vi "superimpose_test.vi"() -> ()   [LabVIEW 2017]
uses:
  Vision.lvlib
panel:
  out "Image 2":T1(plugin-control)
  in  "Top Image":path=path "C:/Users/Caleb/Desktop/obama.jpg"
  in  "Y":i32=40
  in  "X":i32=20
  in  "Bottom Image":path=path "C:/Users/Caleb/Desktop/Screenshot 2021-05-22 162436.png"
  out "error out":errorcluster
  out "Image":T1(plugin-control)
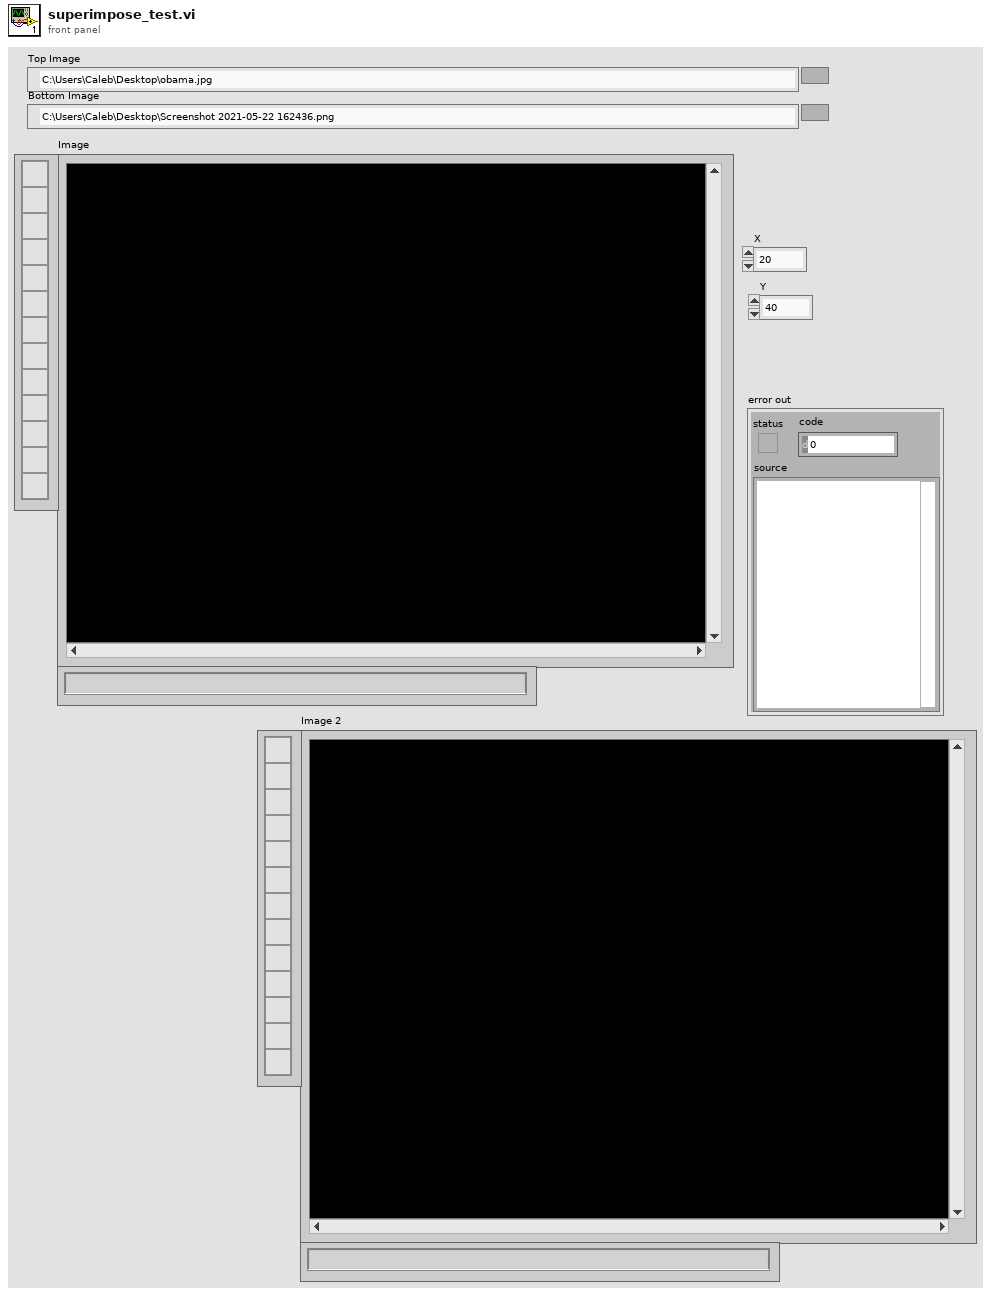
[diagram p1: front panel]
types:
  T1 = typedef "IMAQ Image.ctl" = refnum<image>
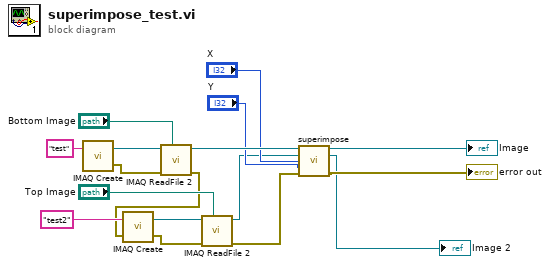
[diagram p0: block diagram]
diagram:
  n1 = call "IMAQ Create"("Image Name"="test") -> ("New Image"=w17:T1, "error out"=w15:errorcluster)  [unwired: 4 in]
  n2 = call "IMAQ ReadFile 2"("File Path"="Bottom Image", "error in (no error)"=w15, "Image"=w17) -> ("error out"=w5:errorcluster, "Image Out"=w13:T1)  [unwired: 4 in, 3 out]
  n3 = call "IMAQ Create"("Image Name"="test2", "error in (no error)"=w5) -> ("New Image"=w8:T1, "error out"=w4:errorcluster)  [unwired: 3 in]
  n4 = call "IMAQ ReadFile 2"("File Path"="Top Image", "error in (no error)"=w4, "Image"=w8) -> ("error out"=w3:errorcluster, "Image Out"=w2:T1)  [unwired: 4 in, 3 out]
  n5 = call "superimpose.vi"("Bottom Image"=w13, "Top Image"=w2, "X"="X", "Y"="Y", "error in (no error)"=w3) -> ("Bottom Image out"=→"Image":T1, "Top Image out"=→"Image 2":T1, "error out"=→"error out":errorcluster)  [unwired: 8 in]
